vi "myRIO_BRig_RT_dataTrial_Cue1_n.vi"() -> (2 "output_Cue1_n":i32)   [LabVIEW 2014]
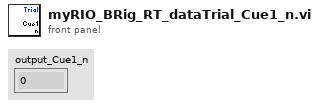
[diagram p1: front panel]
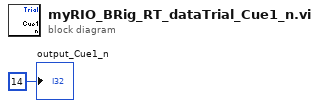
[diagram p0: block diagram]
diagram:
  "output_Cue1_n" <- 14 ("output_iBlock")
